vi "Send error.vi"(8 "error in (no error)":errorcluster, 10 "Error":errorcluster, 11 "Unregister JSON in":refnum<class "Unregister JSON.lvclass">) -> (0 "error out":errorcluster, 3 "Unregister JSON out":refnum<class "Unregister JSON.lvclass">)   [LabVIEW 2020, in "wamplv.lvlib" / "Unregister JSON.lvclass"]
uses:
  Unregister JSON.lvclass
  Unregister JSON.lvclass/Unregister JSON.ctl
  WAMP Client/API/TypeDefs/Error or abort detail (JSON).ctl
  wamplv.lvlib
  WAMP Client/Private/TypeDef/Success or error (JSON).ctl
panel:
  in  "Unregister result":T1={"Success?"=FALSE, "URI"="", "Error/Abort details (JSON)"={"URI"="", "Arguments Payload"="", "ArgumentKw Payload"="{}", "Details"="{}", "Associated LabVIEW Error"={"status"=FALSE, "code"=0, "source"=""}}}
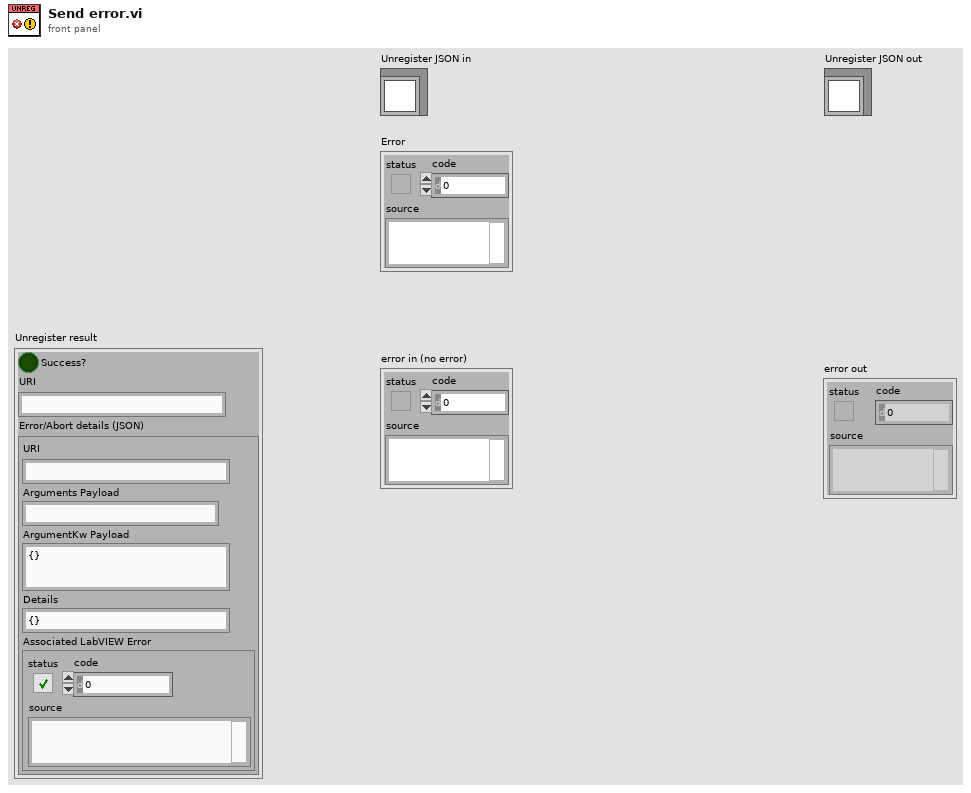
[diagram p1: front panel]
types:
  T1 = typedef "wamplv.lvlib/Success or error (JSON).ctl" = cluster{"Success?":bool, "URI":string, "Error/Abort details (JSON)":T2}
  T2 = typedef "wamplv.lvlib/Error or abort detail (JSON).ctl" = cluster{"URI":string, "Arguments Payload":string, "ArgumentKw Payload":string, "Details":string, "Associated LabVIEW Error":errorcluster}
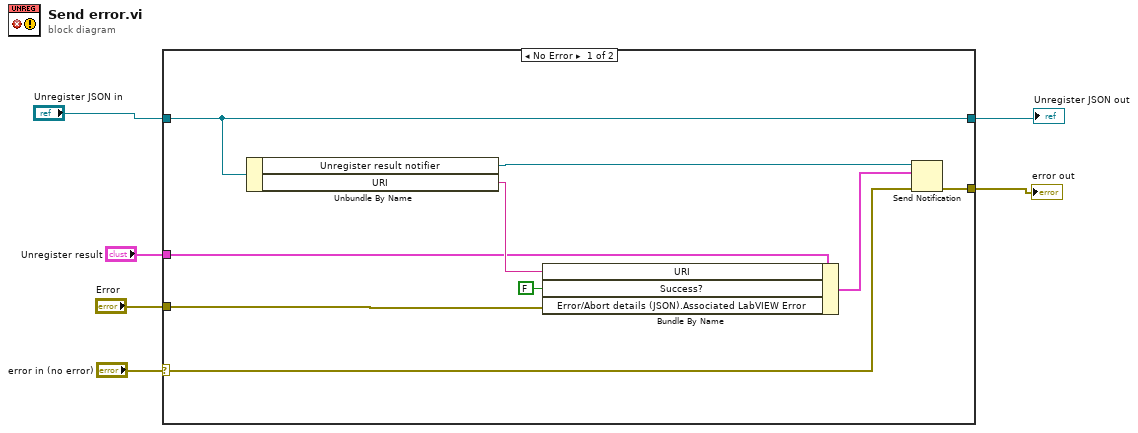
[diagram p0: block diagram]
diagram:
  n1 = case shown="No Error" "error in (no error)" {
    selector: "error in (no error)" -> [w12 w16]
    tunnel: "Unregister JSON in" -> [w10 w17]
    tunnel: [w11 w16] -> w2
    tunnel: [w10 w17] -> w4
    tunnel: "Unregister result" -> [w9 _]
    tunnel: "Error" -> [w8 _]
    frame No Error {
      n2 = Unbundle By Name(w10) -> ("Unregister result notifier"=w15:refnum<notifier>, "URI"=w14:string)
      n3 = Bundle By Name(cluster=w9, "URI"=w14, "Success?"=FALSE, "Error/Abort details (JSON).Associated LabVIEW Error"=w8) -> (w13:T1)
      n4 = Send Notification(notification=w13, notifier=w15, error in (no error)=w12) -> (error out=w11:errorcluster)  [unwired: 1 out]
    }
    frame Error {
    }
  }
  "error out" <- w2
  "Unregister JSON out" <- w4
